vi "Process Data.vi"(0 "Stop Processing?":bool, 1 "Processing Configuration":T1 {"Test Parameters"."Allowed Tolerance (%) FS" format="%#_4g"}, 2 "Queue A - Processing":refnum<queue>, 3 "Database":refnum<queue>, 4 "UI":refnum<queue>, 5 "error in (no error)":errorcluster) -> (14 "Stop Processing?":bool, 19 "error out":errorcluster)   [LabVIEW 2026, in "Processing_Engine.lvlib"]
doc: "This VI uses the TDMS Write function to write data to a TDMS file."
uses:
  Processing_Engine.lvlib
  Processing Settings.ctl
  controls/Messaging Payloads/Sensor CoreData.ctl
  controls/Messaging Payloads/Sensor CoreData Cluster.ctl
  controls/UI/Units Enum.ctl
  controls/UI/Signal Enum.ctl
  Test Parameters.ctl
  Test Parameters Cluster.ctl
  controls/UI/Measurement Role.ctl
  controls/UI/Test Sequence Context.ctl
  controls/UI/Direction.ctl
  support/Architecture/Message Queue/Message Cluster.ctl
  controls/Messaging Payloads/Processed Calibration Point.ctl
  Test Status.ctl
  controls/UI/Test Sequence Enum.ctl
  support/Architecture/Message Queue/Enqueue Message (Single).vi
  support/Architecture/Message Queue/Message Queue.lvlib
  Settings/Settings.lvlib
  Analysis/Analysis.lvlib
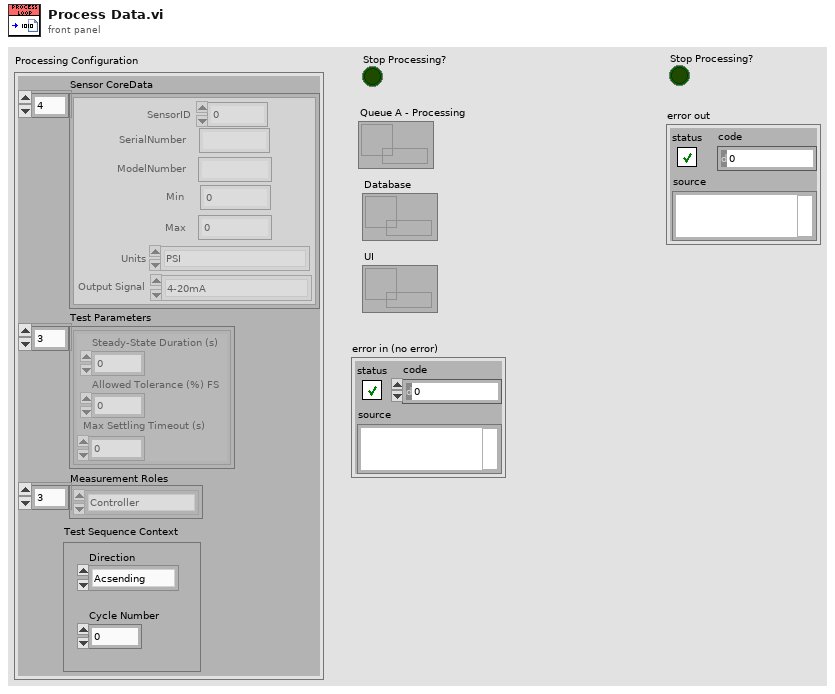
[diagram p1: front panel]
types:
  T1 = typedef "Processing_Engine.lvlib/Processing Settings.ctl" = cluster{"Sensor CoreData":T2, "Test Parameters":T6, "Measurement Roles":T8[], "Test Sequence Context":T9}
  T2 = typedef "Sensor CoreData.ctl" = T3[]
  T3 = typedef "Settings.lvlib/Sensor CoreData Cluster.ctl" = cluster{"SerialNumber":string, "ModelNumber":string, "Min":dbl, "Max":dbl, "Units":T4, "Output Signal":T5, "SensorID":i32}
  T4 = typedef "Units Enum.ctl" = enum16{"PSI", "Deg C", "kPa", "GPM"}
  T5 = typedef "Signal Enum.ctl" = enum16{"4-20mA", "0-10V", "Thermocouple Type K"}
  T6 = typedef "Processing_Engine.lvlib/Test Parameters.ctl" = T7[]
  T7 = typedef "Settings.lvlib/Test Parameters Cluster.ctl" = cluster{"Steady-State Duration (s)":i32, "Allowed Tolerance (%) FS":dbl, "Max Settling Timeout (s)":i32}
  T8 = typedef "Settings.lvlib/Measurement Role.ctl" = enum16{"Controller", "Reference", "UUT", "Disable", "All"}
  T9 = typedef "Settings.lvlib/Test Sequence Context.ctl" = cluster{"Direction":T10, "Cycle Number":i32}
  T10 = typedef "Settings.lvlib/Direction.ctl" = enum16{"Acsending", "Descending"}
  T11 = typedef "Test Sequence Enum.ctl" = enum16{"Idle", "Start Point", "Point Complete", "Test Complete", "Abort Test", "Reset"}
  T12 = typedef "Processed Calibration Point.ctl" = cluster{"Reference Value":dbl, "Measured Value":dbl, "Error":dbl, "Pass/Fail":bool, "Setpoint":dbl, "Cycle Number":i32, "Direction":T10, "Test Status":T13}
  T13 = typedef "Analysis.lvlib/Test Status.ctl" = enum16{"Overall Pass", "Overall Fail", "Test Running"}
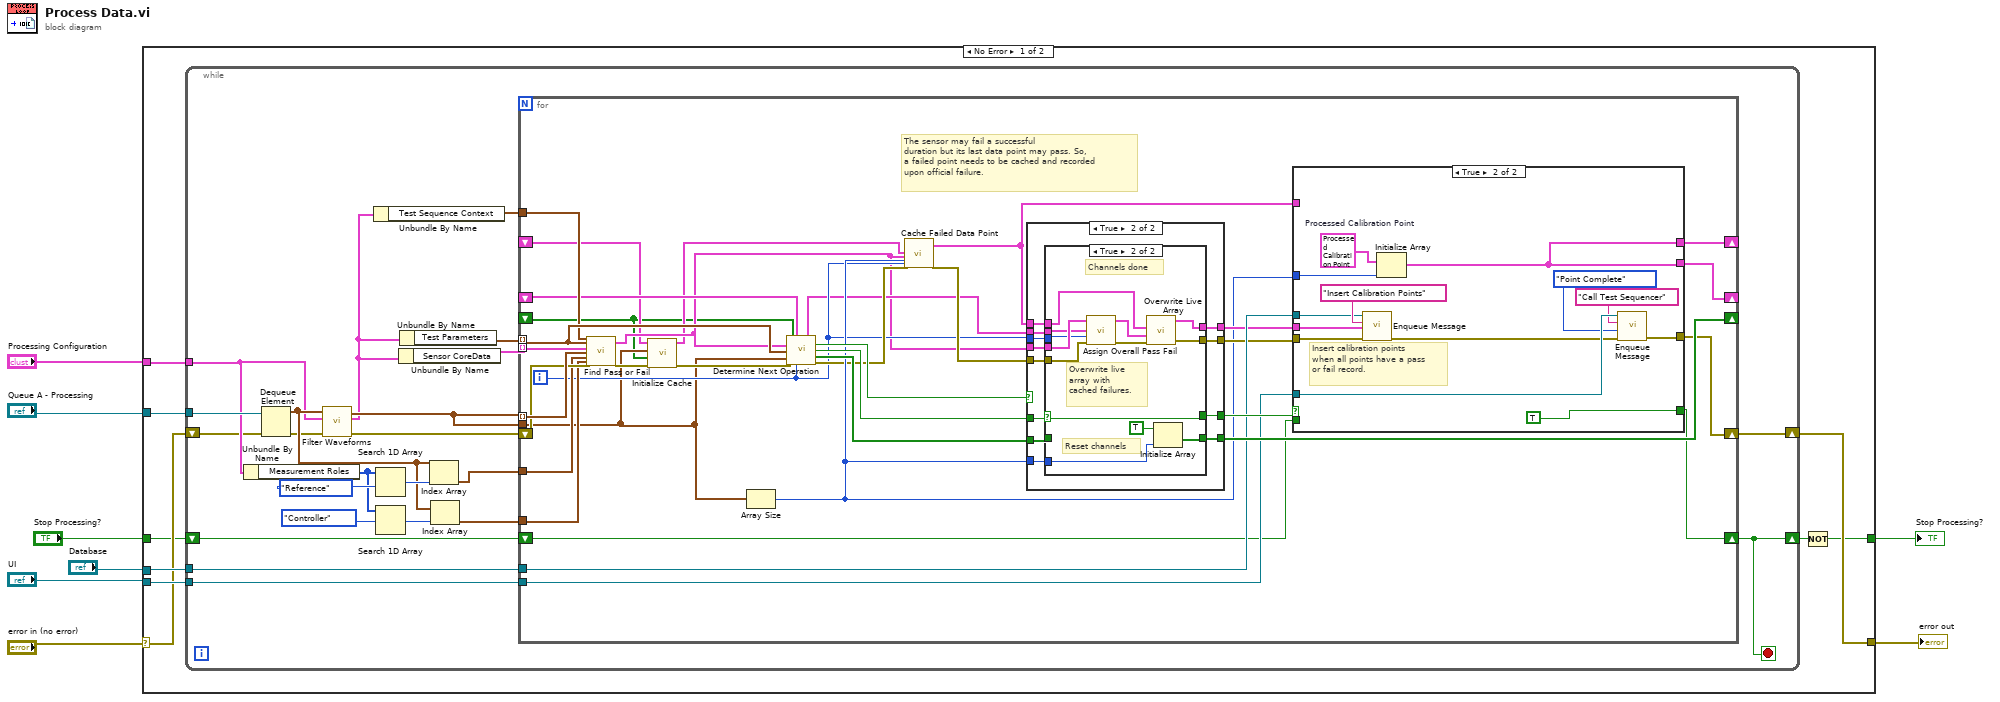
[diagram p0: block diagram]
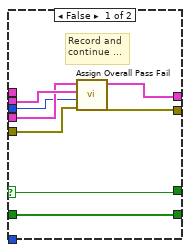
[diagram p4: hidden frame]
diagram:
  n1 = case shown="No Error" "error in (no error)" {
    selector: "error in (no error)" -> [w12 w131]
    tunnel: "Processing Configuration" -> [w13 _]
    tunnel: "Database" -> [w16 _]
    tunnel: [w15 w131] -> w4
    tunnel: "Queue A - Processing" -> [w17 _]
    tunnel: "UI" -> [w14 _]
    tunnel: "Stop Processing?" -> [w11 w130]
    tunnel: [w9 w130] -> w1
    frame No Error {
      n2 = while {
        tunnel: w17 -> [w40]
        tunnel: w16 -> [w39]
        tunnel: w14 -> [w28]
        tunnel: w13 -> [w23]
        shift-right: [w29] -> w15
        shift-left: w12 -> [w22]
        shift-right: [w18] -> w10
        shift-left: w11 -> [w19]
        stop <- w18 stop-if-true
        n3 = Unbundle By Name(w23) -> ("Measurement Roles"=w33:T8[])
        n4 = Dequeue Element(queue=w40, error in (no error)=w22) -> (element=w24:waveform(dbl)[], error out=w21:errorcluster)  [unwired: 1 in, 2 out]
        n5 = call "Filter Waveforms.vi"("error in (no error)"=w21, "Processing Configuration"=w23, "All Waveforms"=w24) -> ("error out"=w25:errorcluster, "Filtered Processing Configuration"=w20:T1, "UUT Waveforms"=w26:waveform(dbl)[])  [unwired: 6 in]
        n6 = Unbundle By Name(w20) -> ("Test Sequence Context"=w27:T9)
        n7 = Search 1D Array(1D array=w33, element=Measurement_Role."Reference") -> (index of element=w35:i32)  [unwired: 1 in]
        n8 = Search 1D Array(1D array=w33, element=Measurement_Role."Controller") -> (index of element=w31:i32)  [unwired: 1 in]
        n9 = Unbundle By Name(w20) -> ("Sensor CoreData"=w37:T2)
        n10 = Unbundle By Name(w20) -> ("Test Parameters"=w38:T6)
        n11 = Index Array(array=w24, index=w35) -> (element=w34:waveform(dbl))
        n12 = Index Array(array=w24, index=w31) -> (element=w30:waveform(dbl))
        n13 = for {
          tunnel: w26 -> [w75] mode=indexing
          tunnel: w38 -> [w62] mode=indexing
          tunnel: w37 -> [w74] mode=indexing
          shift-right: [w73] -> _
          shift-left: _ -> [w43]
          shift-right: [w70] -> w29
          shift-left: w25 -> [w63]
          shift-right: [w54] -> _
          shift-left: _ -> [w51]
          tunnel: w39 -> [w69]
          shift-right: [w52] -> _
          shift-left: _ -> [w46]
          tunnel: w26 -> [w44]
          tunnel: w34 -> [w61]
          tunnel: w30 -> [w58]
          tunnel: w28 -> [w57]
          tunnel: w27 -> [w56]
          shift-right: [w41] -> w18
          shift-left: w19 -> [w42]
          i -> [w55]
          # "The sensor may fail a successful \nduration but its last data point may pass. So,\na failed point needs to be cached and recorded\nupon official failure."
          n14 = call "Find Pass or Fail.vi"("Test Sequence Context"=w56, "Test Parameters"=w62, "Sensor CoreData"=w74, "UUT Waveform"=w75, "Reference Waveform"=w61, "Setpoint Waveform"=w58, "error in (no error)"=w63) -> ("New Processed Calibration Point"=w49:T12, "error out"=w48:errorcluster)  [unwired: 19 in]
          n15 = call "Initialize Cache.vi"("error in (no error)"=w48, "Initialized Array in"=w43, "Array in"=w44, "Current Cache in"=w46) -> ("error out"=w47:errorcluster, "Current Cache out"=w45:T12[])  [unwired: 6 in]
          n16 = Array Size(array=w44) -> (size(s)=w64:i32)
          n17 = call "Determine Next Operation.vi"("Initialize Array in"=w43, "Record Array in"=w51, "Processed Calibration Point"=w49, "Test Parameters"=w62, "Array in"=w44, "error in (no error)"=w47, "Array Index or Channel"=w55) -> ("Record Array out"=w50:T12[], "Record?"=w65:bool, "Done?"=w66:bool, "Recorded Channels"=w72:bool[], "error out"=w60:errorcluster)  [unwired: 3 in, 1 out]
          n18 = call "Cache Failed Data Point.vi"("Current Cache"=w45, "New Cache"=w49, "Channels Size"=w64, "Channel Index"=w55, "error in (no error)"=w60) -> ("Cache out"=w53:T12[], "error out"=w59:errorcluster)  [unwired: 21 in]
          n19 = case shown="True" w65 {
            tunnel: w66 -> [w95 w108]
            tunnel: [w95 w107] -> w71
            tunnel: [w94 w106] -> w73
            tunnel: w72 -> [w94 w105]
            tunnel: w64 -> [_ w104]
            tunnel: w49 -> [_ w101]
            tunnel: w50 -> [w96 w103]
            tunnel: w55 -> [_ w102]
            tunnel: [w96 w100] -> w68
            tunnel: w53 -> [_ w99]
            tunnel: w59 -> [w93 w98]
            tunnel: [w93 w97] -> w67
            frame False {
              # "Don't record."
            }
            frame True {
              n20 = case shown="True" w108 {
                selector: w108 -> [w116 w126]
                tunnel: w105 -> [w115 _]
                tunnel: [w116 w126] -> w107
                tunnel: [w115 w128] -> w106
                tunnel: w104 -> [_ w127]
                tunnel: w103 -> [w114 w123]
                tunnel: w102 -> [w112 w120]
                tunnel: w101 -> [w113 w124]
                tunnel: [w109 w117] -> w100
                tunnel: w99 -> [_ w119]
                tunnel: w98 -> [w111 w122]
                tunnel: [w110 w125] -> w97
                frame False {
                  # "Record and\ncontinue ..."
                  n21 = call "Assign Overall Pass Fail.vi"("error in (no error)"=w111, "Channel"=w112, "Record Array in"=w114, "New Processed Calibration Point in"=w113) -> ("error out"=w110:errorcluster, "Record Array out"=w109:T12[])  [unwired: 6 in]
                }
                frame True {
                  # "Overwrite live\narray with \ncached failures."
                  # "Channels done"
                  # "Reset channels"
                  n22 = call "Assign Overall Pass Fail.vi"("error in (no error)"=w122, "Channel"=w120, "Record Array in"=w123, "New Processed Calibration Point in"=w124) -> ("error out"=w121:errorcluster, "Record Array out"=w118:T12[])  [unwired: 6 in]
                  n23 = call "Overwrite Live Array.vi"("error in (no error)"=w121, "Live Array"=w118, "Cache Array"=w119) -> ("error out"=w125:errorcluster, "Record Array"=w117:T12[])  [unwired: 7 in]
                  n24 = Initialize Array(TRUE ("Record?"), w127) -> (w128:bool[])
                }
              }
            }
          }
          n25 = case shown="True" w71 {
            tunnel: w69 -> [_ w91]
            tunnel: w67 -> [w79 w90]
            tunnel: [w79 w81] -> w70
            tunnel: [w78 w83] -> w54
            tunnel: w68 -> [w78 w89]
            tunnel: w64 -> [_ w87]
            tunnel: w57 -> [_ w86]
            tunnel: w53 -> [w77 _]
            tunnel: [w77 w83] -> w52
            tunnel: [w76 TRUE] -> w41
            tunnel: w42 -> [w76 _]
            frame False {
            }
            frame True {
              w88 = T12 {"Reference Value"=0.0, "Measured Value"=0.0, "Error"=0.0, "Pass/Fail"=TRUE, "Setpoint"=0.0, "Cycle Number"=0, "Direction"=enum."Acsending", "Test Status"=enum."Overall Fail"}  # Processed Calibration Point
              # "Insert calibration points\nwhen all points have a pass\nor fail record."
              n26 = call-poly "Enqueue Message.vi"("error in (no error)"=w90, "Message Data"=w89, "Message"="Insert Calibration Points", "Message Queue"=w91) -> ("error out"=w80:errorcluster)  [unwired: 6 in, 1 out]
              n27 = Initialize Array(w88, w87) -> (w83:T12[])
              n28 = call-poly "Enqueue Message.vi"("error in (no error)"=w80, "Message Data"=Test_Sequence_Enum."Point Complete" ("Test Sequence Enum"), "Message"="Call Test Sequencer", "Message Queue"=w86) -> ("error out"=w81:errorcluster)  [unwired: 6 in, 1 out]
            }
          }
        }
      }
      n29 = Not(x=w10) -> (.not. x?=w9:bool)
    }
    frame Error {
    }
  }
  "error out" <- w4
  "Stop Processing?" <- w1
